vi "0_Waveform_Anomaly_Detection(Dataset_Generation).vi"() -> ()   [LabVIEW 2020]
uses:
  <vilib>/Utility/file.llb/Write Delimited Spreadsheet (DBL).vi
panel:
  in  "Validation portion (%)":u32=5
  in  "Train Dataset Folder Path":path=path "D:/working/Anomaly Detection/Train"
  in  "Number of Dataset Samples(Test)":u32=500
  in  "Number of Dataset Samples(Train)":i32=10000
  in  "Validation Dataset Folder Path":path=path "D:/working/Anomaly Detection/Validation"
  in  "Test Dataset Folder Path":path=path "D:/working/Anomaly Detection/Test"
  in  "sampling info":cluster{"Fs":dbl, "#s":dbl}={"Fs"=10000.0, "#s"=2000.0}
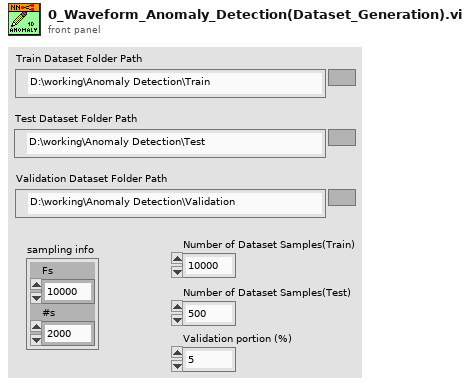
[diagram p1: front panel]
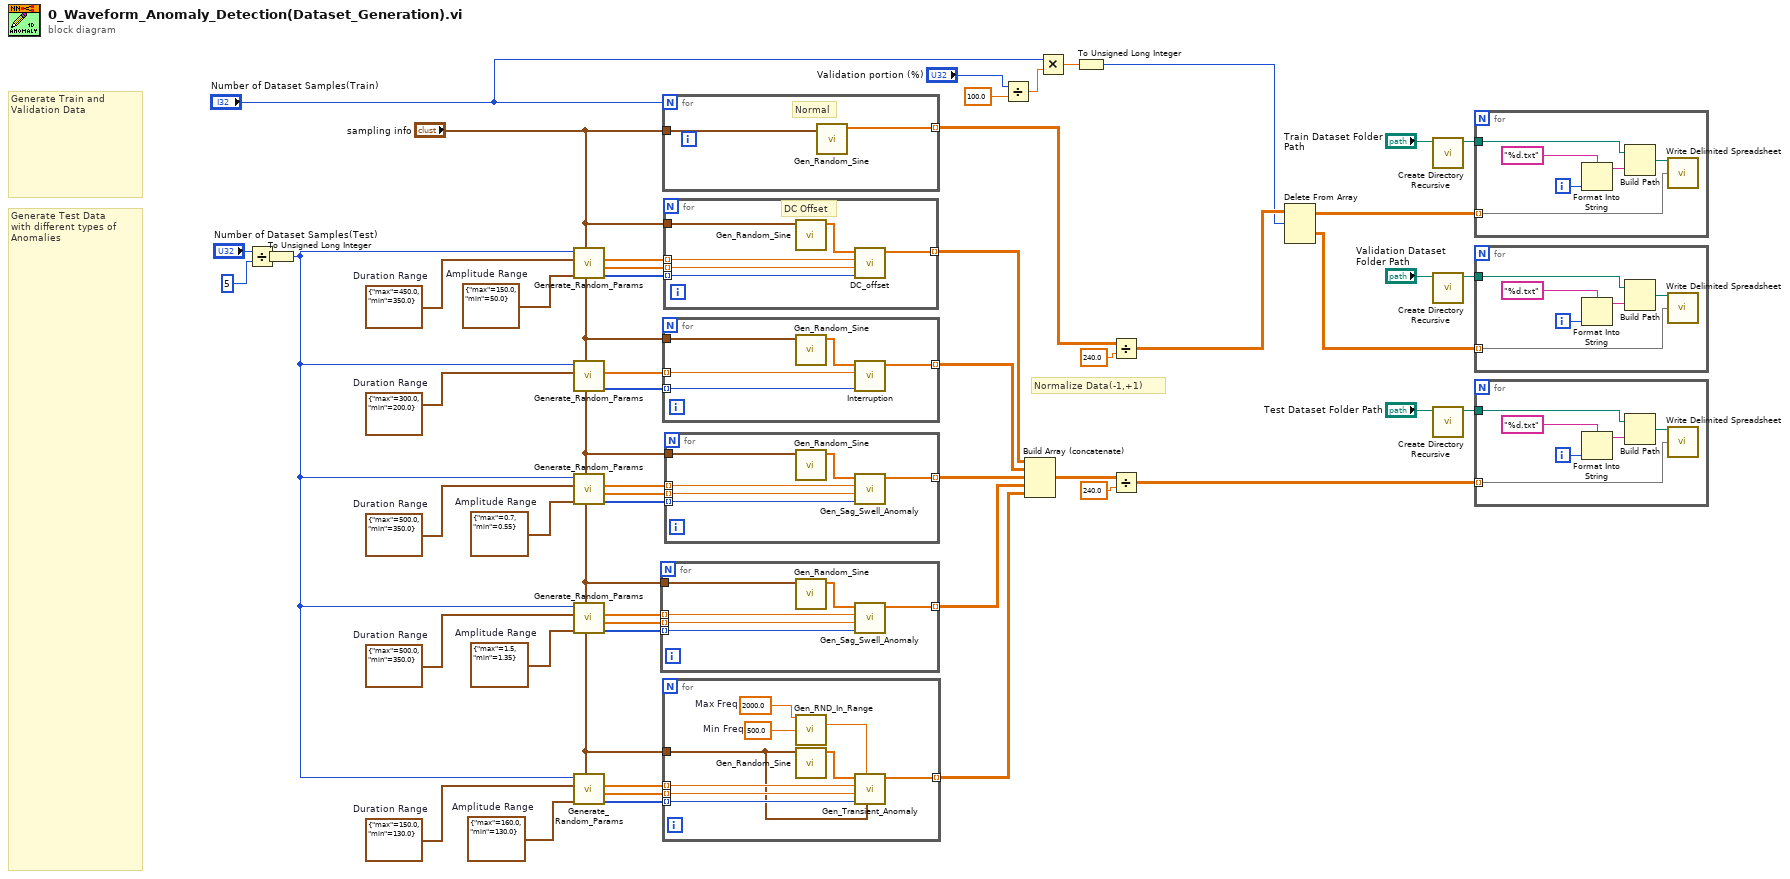
[diagram p0: block diagram]
diagram:
  w32 = cluster{"max":dbl, "min":dbl} {"max"=150.0, "min"=130.0}  # Duration Range
  w33 = cluster{"max":dbl, "min":dbl} {"max"=160.0, "min"=130.0}  # Amplitude Range
  w38 = cluster{"max":dbl, "min":dbl} {"max"=500.0, "min"=350.0}  # Duration Range
  w37 = cluster{"max":dbl, "min":dbl} {"max"=1.5, "min"=1.35}  # Amplitude Range
  w42 = cluster{"max":dbl, "min":dbl} {"max"=500.0, "min"=350.0}  # Duration Range
  w43 = cluster{"max":dbl, "min":dbl} {"max"=0.7, "min"=0.55}  # Amplitude Range
  w46 = cluster{"max":dbl, "min":dbl} {"max"=300.0, "min"=200.0}  # Duration Range
  w47 = cluster{"max":dbl, "min":dbl} {"max"=450.0, "min"=350.0}  # Duration Range
  w48 = cluster{"max":dbl, "min":dbl} {"max"=150.0, "min"=50.0}  # Amplitude Range
  # "Generate Test Data\nwith different types of Anomalies"
  # "Generate Train and Validation Data"
  # "Normalize Data(-1,+1)"
  n1 = Divide(x="Number of Dataset Samples(Test)", y=5) -> (x/y=w14:dbl)
  n2 = To Unsigned Long Integer(number=w14) -> (unsigned 32bit integer=w11:u32)
  n3 = call "Generate_Random_Params.vi"("sampling info"="sampling info", "Amplitude Range"=w48, "Duration Range"=w47, "Dataset Samples"=w11) -> ("Duration"=w49:i32[], "Amplitude"=w50:sgl[], "Position"=w51:dbl[])  [unwired: 5 in]
  n4 = call "Generate_Random_Params.vi"("sampling info"="sampling info", "Duration Range"=w46, "Dataset Samples"=w11) -> ("Duration"=w44:i32[], "Position"=w45:dbl[])  [unwired: 6 in, 1 out]
  n5 = call "Generate_Random_Params.vi"("sampling info"="sampling info", "Amplitude Range"=w43, "Duration Range"=w42, "Dataset Samples"=w11) -> ("Duration"=w39:i32[], "Amplitude"=w40:sgl[], "Position"=w41:dbl[])  [unwired: 5 in]
  n6 = call "Generate_Random_Params.vi"("sampling info"="sampling info", "Amplitude Range"=w37, "Duration Range"=w38, "Dataset Samples"=w11) -> ("Duration"=w34:i32[], "Amplitude"=w35:sgl[], "Position"=w36:dbl[])  [unwired: 5 in]
  n7 = call "Generate_Random_Params.vi"("sampling info"="sampling info", "Amplitude Range"=w33, "Duration Range"=w32, "Dataset Samples"=w11) -> ("Duration"=w29:i32[], "Amplitude"=w30:sgl[], "Position"=w31:dbl[])  [unwired: 5 in]
  n8 = for {
    tunnel: [w58] -> w21 mode=indexing
    tunnel: w36 -> [w57] mode=indexing
    tunnel: w35 -> [w56] mode=indexing
    tunnel: w34 -> [w55] mode=indexing
    tunnel: "sampling info" -> [w54]
    n9 = call "Gen_Random_Sine.vi"("sampling info"=w54) -> ("data"=w59:sgl[])  [unwired: 10 in]
    n10 = call "Gen_Sag_Swell_Anomaly.vi"("Duration"=w55, "Amplitude"=w56, "Position"=w57, "Sine"=w59) -> ("Sine+Anomaly"=w58:sgl[])  [unwired: 7 in]
  }
  n11 = for {
    N: "Number of Dataset Samples(Train)" -> [_]
    tunnel: [w61] -> w22 mode=indexing
    tunnel: "sampling info" -> [w60]
    # "Normal"
    n12 = call "Gen_Random_Sine.vi"("sampling info"=w60) -> ("data"=w61:sgl[])  [unwired: 10 in]
  }
  n13 = for {
    tunnel: [w66] -> w27 mode=indexing
    tunnel: w45 -> [w64] mode=indexing
    tunnel: w44 -> [w63] mode=indexing
    tunnel: "sampling info" -> [w62]
    n14 = call "Gen_Random_Sine.vi"("sampling info"=w62) -> ("data"=w65:sgl[])  [unwired: 10 in]
    n15 = call "Interruption.vi"("Duration"=w63, "Position"=w64, "Sine"=w65) -> ("Sine+Anomaly"=w66:sgl[])  [unwired: 8 in]
  }
  n16 = for {
    tunnel: [w74] -> w26 mode=indexing
    tunnel: w31 -> [w70] mode=indexing
    tunnel: w30 -> [w69] mode=indexing
    tunnel: w29 -> [w68] mode=indexing
    tunnel: "sampling info" -> [w67]
    w71 = 2000.0  # Max Freq
    w72 = 500.0  # Min Freq
    n17 = call "Gen_RND_In_Range.vi"("Upper Bound"=w71, "Lower Bound"=w72) -> ("RND_In_Range"=w73:dbl)  [unwired: 13 in]
    n18 = call "Gen_Random_Sine.vi"("sampling info"=w67) -> ("data"=w75:sgl[])  [unwired: 10 in]
    n19 = call "Gen_Transient_Anomaly.vi"("sampling info"=w67, "Frequency"=w73, "Tau"=w68, "Amplitude"=w69, "Position"=w70, "Sine"=w75) -> ("Sine+Anomaly"=w74:sgl[])  [unwired: 5 in]
  }
  n20 = for {
    tunnel: [w80] -> w28 mode=indexing
    tunnel: w51 -> [w79] mode=indexing
    tunnel: w50 -> [w78] mode=indexing
    tunnel: w49 -> [w77] mode=indexing
    tunnel: "sampling info" -> [w76]
    # "DC Offset"
    n21 = call "Gen_Random_Sine.vi"("sampling info"=w76) -> ("data"=w81:sgl[])  [unwired: 10 in]
    n22 = call "DC_offset.vi"("Duration"=w77, "Ampltude"=w78, "Position"=w79, "Sine"=w81) -> ("Sine+Anomaly"=w80:sgl[])  [unwired: 7 in]
  }
  n23 = for {
    tunnel: [w86] -> w24 mode=indexing
    tunnel: w41 -> [w85] mode=indexing
    tunnel: w40 -> [w84] mode=indexing
    tunnel: w39 -> [w83] mode=indexing
    tunnel: "sampling info" -> [w82]
    n24 = call "Gen_Random_Sine.vi"("sampling info"=w82) -> ("data"=w87:sgl[])  [unwired: 10 in]
    n25 = call "Gen_Sag_Swell_Anomaly.vi"("Duration"=w83, "Amplitude"=w84, "Position"=w85, "Sine"=w87) -> ("Sine+Anomaly"=w86:sgl[])  [unwired: 7 in]
  }
  n26 = Divide(x="Validation portion (%)", y=100.0) -> (x/y=w5:dbl)
  n27 = Build Array (concatenate)(w28, w27, w24, w21, w26) -> (w23:sgl[][])
  n28 = Multiply(x="Number of Dataset Samples(Train)", y=w5) -> (x*y=w4:dbl)
  n29 = To Unsigned Long Integer(number=w4) -> (unsigned 32bit integer=w3:u32)
  n30 = Divide(x=w22, y=sgl 240.0) -> (x/y=w12:sgl[][])
  n31 = Divide(x=w23, y=sgl 240.0) -> (x/y=w18:sgl[][])
  n32 = Delete From Array(array=w12, length=w3) -> (deleted portion=w2:sgl[][], array with subset deleted=w1:sgl[][])  [unwired: 2 in]
  n33 = call <vilib>:"Create Directory Recursive.vi"("directory"="Train Dataset Folder Path") -> ("directory copy"=w9:path)  [unwired: 4 in, 2 out]
  n34 = call <vilib>:"Create Directory Recursive.vi"("directory"="Validation Dataset Folder Path") -> ("directory copy"=w16:path)  [unwired: 4 in, 2 out]
  n35 = call <vilib>:"Create Directory Recursive.vi"("directory"="Test Dataset Folder Path") -> ("directory copy"=w17:path)  [unwired: 4 in, 2 out]
  n36 = for {
    tunnel: w1 -> [w92] mode=indexing
    tunnel: w9 -> [w93]
    i -> [w89]
    n37 = Format Into String(format string="%d.txt", w89) -> (resulting string=w88:string)  [unwired: 2 in, 1 out]
    n38 = Build Path(base path=w93, name or relative path=w88) -> (appended path=w91:path)
    n39 = call-poly <vilib>:"Write Delimited Spreadsheet.vi"("file path (dialog if empty)"=w91, "1D data"=w92) -> ()  [unwired: 12 in, 2 out]
  }
  n40 = for {
    tunnel: w2 -> [w98] mode=indexing
    tunnel: w16 -> [w99]
    i -> [w95]
    n41 = Format Into String(format string="%d.txt", w95) -> (resulting string=w94:string)  [unwired: 2 in, 1 out]
    n42 = Build Path(base path=w99, name or relative path=w94) -> (appended path=w97:path)
    n43 = call-poly <vilib>:"Write Delimited Spreadsheet.vi"("file path (dialog if empty)"=w97, "1D data"=w98) -> ()  [unwired: 12 in, 2 out]
  }
  n44 = for {
    tunnel: w18 -> [w104] mode=indexing
    tunnel: w17 -> [w105]
    i -> [w101]
    n45 = Format Into String(format string="%d.txt", w101) -> (resulting string=w100:string)  [unwired: 2 in, 1 out]
    n46 = Build Path(base path=w105, name or relative path=w100) -> (appended path=w103:path)
    n47 = call-poly <vilib>:"Write Delimited Spreadsheet.vi"("file path (dialog if empty)"=w103, "1D data"=w104) -> ()  [unwired: 12 in, 2 out]
  }
